vi "_035.vi"() -> ()   [LabVIEW 2024]
panel:
  in  "Stop Button":bool
  out "D":dbl
  in  "Numeric 8":dbl
  in  "Numeric 7":dbl
  in  "Div":bool
  out "M":dbl
  in  "Numeric 6":dbl
  in  "Numeric 5":dbl
  in  "Mul":bool
  out "S":dbl
  in  "Numeric 3":dbl
  in  "Numeric 4":dbl
  in  "Sub":bool
  out "A":dbl
  in  "Numeric 2":dbl
  in  "Numeric 1":dbl
  in  "Add":bool
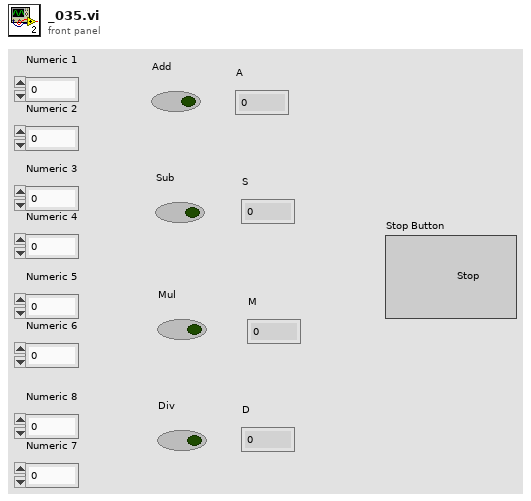
[diagram p1: front panel]
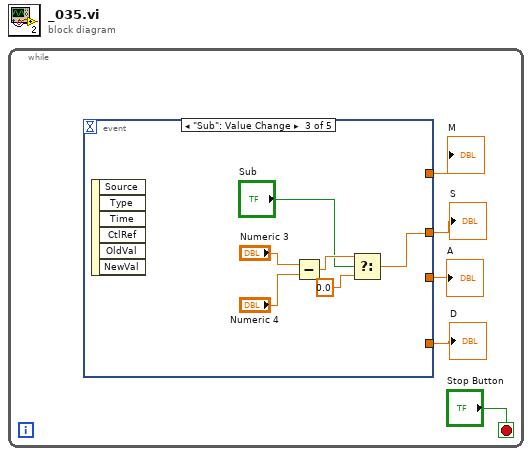
[diagram p0: block diagram]
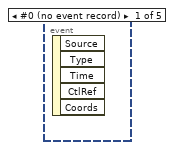
[diagram p2: hidden frame]
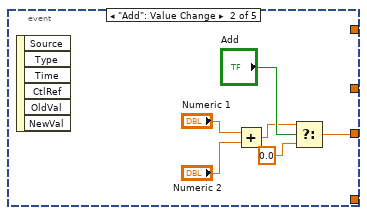
[diagram p3: hidden frame]
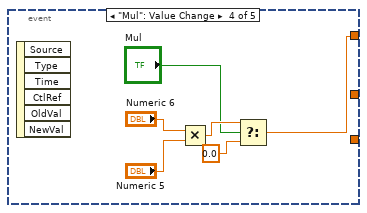
[diagram p4: hidden frame]
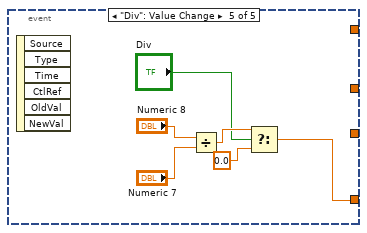
[diagram p5: hidden frame]
diagram:
  n1 = while {
    stop <- "Stop Button" stop-if-true
    n2 = event shown="[2] \"Sub\": Value Change" {
      selector: _ -> [_ _ _ _ _]
      dyn-events: _ -> [_ _ _ _ _]
      timeout: _ -> [_ _ _ _ _]
      tunnel: [_ w6 _ _ _] -> w5
      tunnel: [_ _ w12 _ _] -> w4
      tunnel: [_ _ _ w18 _] -> w3
      tunnel: [_ _ _ _ w24] -> w2
      event #0 (no event record) {
        n3 = event-data() -> ()  [unwired: 1 in, 5 out]
      }
      event "Add": Value Change {
        n4 = event-data() -> ()  [unwired: 1 in, 6 out]
        n5 = Add(x="Numeric 1", y="Numeric 2") -> (x+y=w8:dbl)
        n6 = Select(t=w8, s="Add", f=0.0) -> (s? t:f=w6:dbl)
      }
      event "Sub": Value Change {
        n7 = event-data() -> ()  [unwired: 1 in, 6 out]
        n8 = Subtract(x="Numeric 3", y="Numeric 4") -> (x-y=w15:dbl)
        n9 = Select(t=w15, s="Sub", f=0.0) -> (s? t:f=w12:dbl)
      }
      event "Mul": Value Change {
        n10 = event-data() -> ()  [unwired: 1 in, 6 out]
        n11 = Multiply(x="Numeric 6", y="Numeric 5") -> (x*y=w21:dbl)
        n12 = Select(t=w21, s="Mul", f=0.0) -> (s? t:f=w18:dbl)
      }
      event "Div": Value Change {
        n13 = event-data() -> ()  [unwired: 1 in, 6 out]
        n14 = Divide(x="Numeric 8", y="Numeric 7") -> (x/y=w27:dbl)
        n15 = Select(t=w27, s="Div", f=0.0) -> (s? t:f=w24:dbl)
      }
    }
    "A" <- w5
    "S" <- w4
    "M" <- w3
    "D" <- w2
  }
